vi "FlatToRichhwval_GenericResponse.vi"(5 "OutputClusterType":T1, 11 "InputCluster":T2) -> (3 "OutputCluster":T1)   [LabVIEW 2025, in "OOB gRPC Server.lvlib"]
uses:
  OOB gRPC Server.lvlib
  hwval_GenericResponse_Flat.ctl
  hwval_GenericResponse.ctl
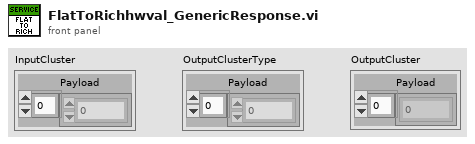
[diagram p1: front panel]
types:
  T1 = typedef "OOB gRPC Server.lvlib/hwval_GenericResponse.ctl" = cluster{"Payload":u8[]}
  T2 = typedef "OOB gRPC Server.lvlib/hwval_GenericResponse_Flat.ctl" = cluster{"Payload":u8[]}
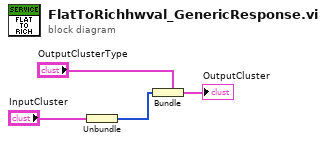
[diagram p0: block diagram]
diagram:
  n1 = Unbundle "Unbundle"("InputCluster") -> ("Payload"=w1:u8[])
  n2 = Bundle "Bundle"(cluster="OutputClusterType", "Payload"=w1) -> (→"OutputCluster":T1)
